vi "displayex.vi"(0 "EncMax":dbl[](array[numeric])=[6.50325, 6.5055000000000005, 6.4670000000000005], 1 "EncPos":cluster{"[0]":dbl, "[1]":dbl, "[2]":dbl}(graph)={"[0]"=1.92575, "[1]"=1.8495000000000001, "[2]"=4.599500000000001} caption="Position", 2 "TargetPos":dbl[](array[numeric])=[3.0, 3.0, 3.0], 3 "Blank":picture, 4 "CurrentState":enum16{"Initialize", "Run", "Finalize"}(ring)=enum."Run", 8 "HoldRange":dbl[](array[numeric])=[3.0, 3.0, 3.0]) -> (5 "Display":picture)   [LabVIEW 2011]
panel:
  in  "DispH":u32=870
  in  "PicRects":T1={"PicTar"={"Index"={"left"=0, "top"=325, "right"=0, "bottom"=525}, "Middle"={"left"=0, "top"=625, "right"=0, "bottom"=825}, "Thumb"={"left"=0, "top"=25, "right"=0, "bottom"=225}}, "PicPos"={"Index"={"left"=0, "top"=325, "right"=0, "bottom"=525}, "Middle"={"left"=0, "top"=625, "right"=0, "bottom"=825}, "Thumb"={"left"=0, "top"=25, "right"=0, "bottom"=225}}}
  in  "PicSizes":T2={"TarHeight"=200, "PosHeight"=200, "TarWidth"=200, "PosWidth"=200}
  in  "DispW":u32=1362
  in  "PosColor":cluster{"Index":u32, "Middle":u32, "Thumb":u32}={"Index"=11372, "Middle"=2113536, "Thumb"=7405568}
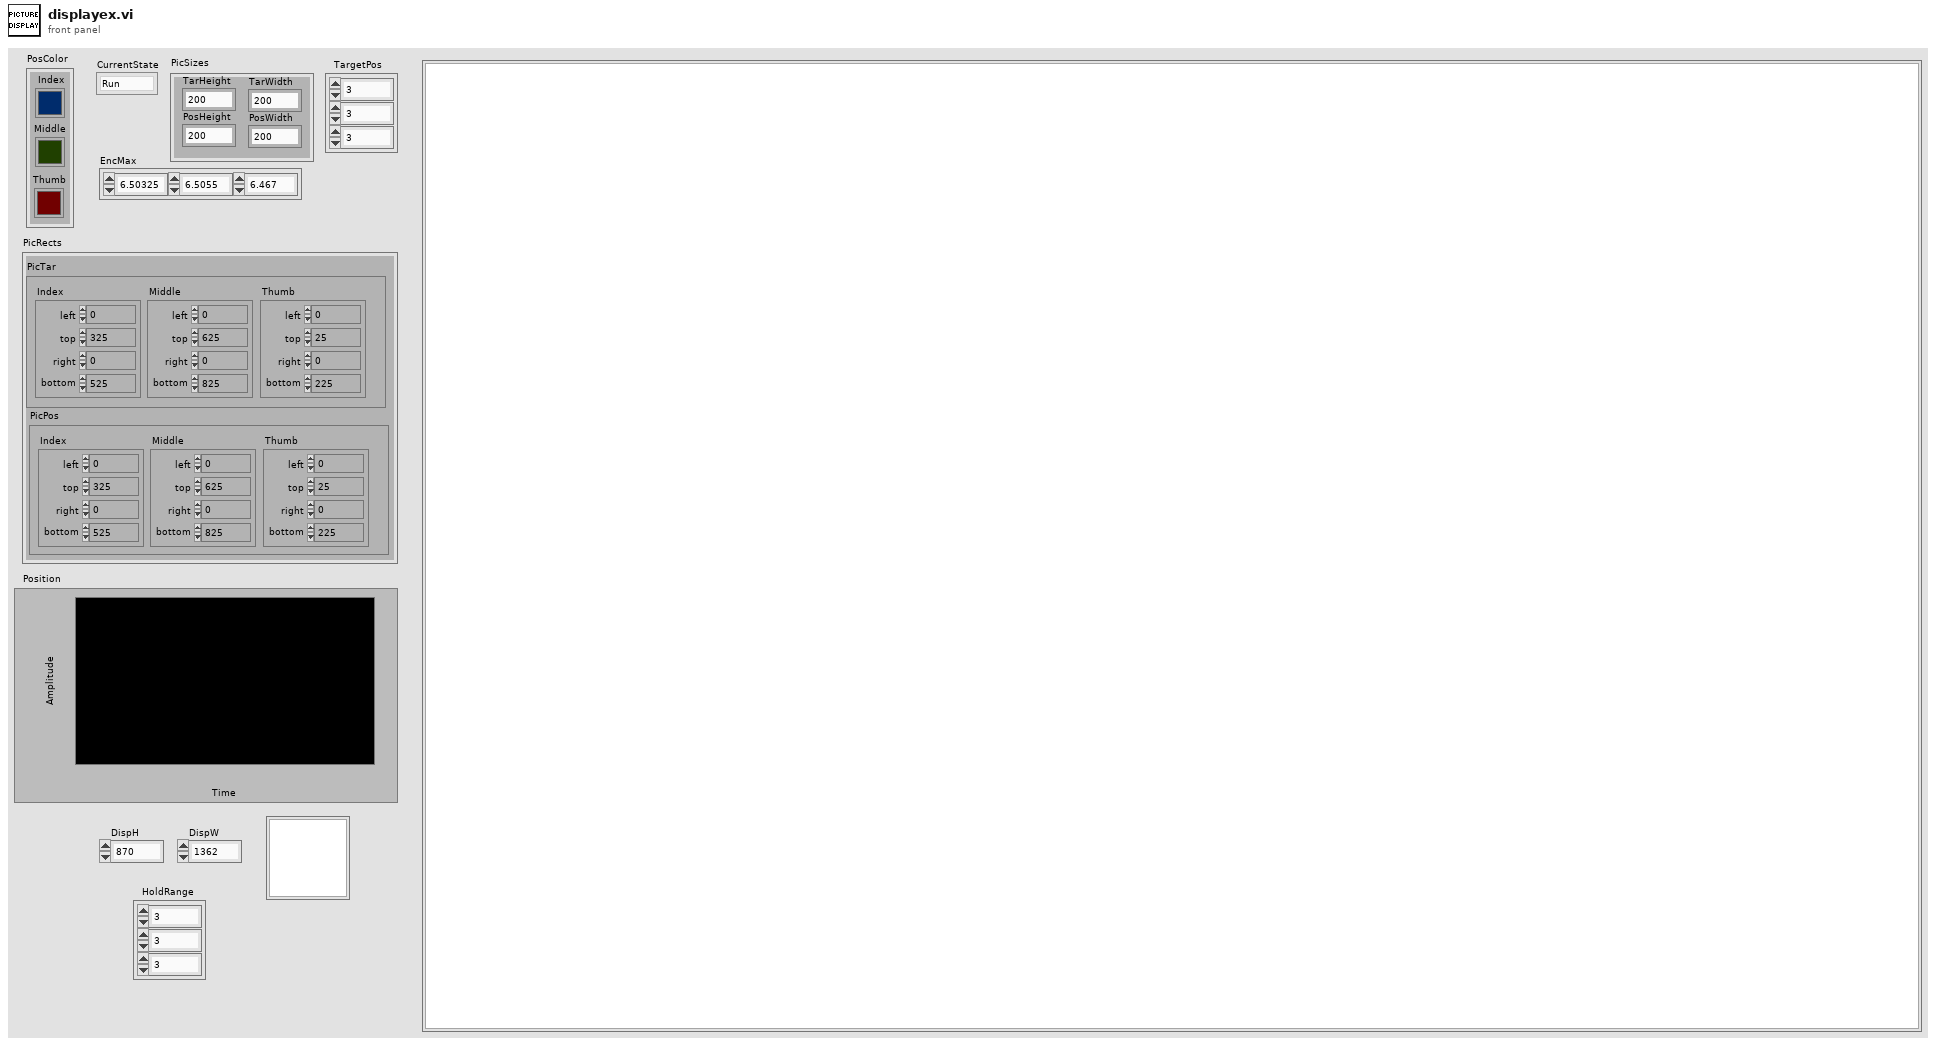
[diagram p1: front panel]
types:
  T1 = cluster{"PicTar":cluster{"Index":cluster{"left":i16, "top":i16, "right":i16, "bottom":i16}, "Middle":cluster{"left":i16, "top":i16, "right":i16, "bottom":i16}, "Thumb":cluster{"left":i16, "top":i16, "right":i16, "bottom":i16}}, "PicPos":cluster{"Index":cluster{"left":i16, "top":i16, "right":i16, "bottom":i16}, "Middle":cluster{"left":i16, "top":i16, "right":i16, "bottom":i16}, "Thumb":cluster{"left":i16, "top":i16, "right":i16, "bottom":i16}}}
  T2 = cluster{"TarHeight":i32, "PosHeight":i32, "TarWidth":i32, "PosWidth":i32}
  T3 = cluster{"Width":u16, "Style":enum32{"Solid", "Dash", "Dot", "DashDot", "DashDotDot"}}
  T4 = typedef "LVBoundsTypeDef.ctl" = cluster{"Width":u32, "Height":u32}
  T5 = cluster{"left":i16, "top":i16, "right":i16, "bottom":i16}
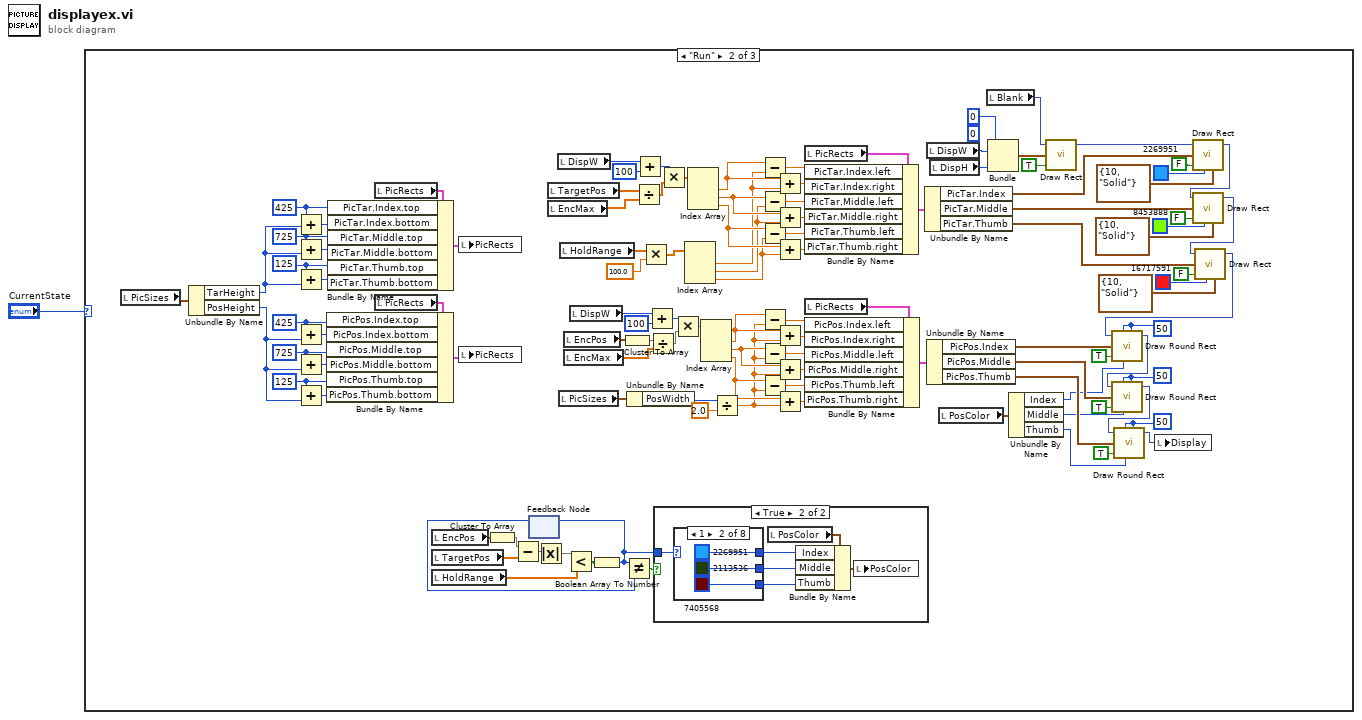
[diagram p0: block diagram]
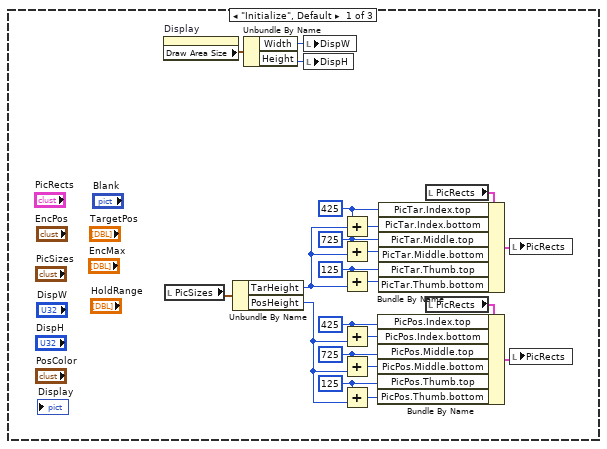
[diagram p2: hidden frame]
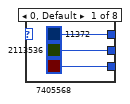
[diagram p4: hidden frame]
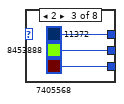
[diagram p5: hidden frame]
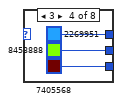
[diagram p6: hidden frame]
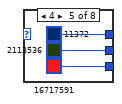
[diagram p7: hidden frame]
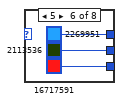
[diagram p8: hidden frame]
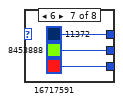
[diagram p9: hidden frame]
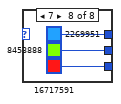
[diagram p10: hidden frame]
diagram:
  n1 = case shown="\"Run\"" "CurrentState" {
    frame "Initialize", Default {
      w15 = 125
      w18 = 725
      w13 = 425
      w11 = 125
      w21 = 725
      w8 = 425
      n2 = property on="Display" class="Pict"() -> ("Draw Area Size"=w4:T4)  [unwired: 2 in, 2 out]
      n3 = local read "PicSizes"() -> (w5:T2)
      n4 = Unbundle By Name(w5) -> ("TarHeight"=w6:i32, "PosHeight"=w7:i32)
      n5 = Unbundle By Name(w4) -> ("Width"=w3:u32, "Height"=w2:u32)
      n6 = local write "DispW"(w3) -> ()
      n7 = local write "DispH"(w2) -> ()
      n8 = Add(x=w13, y=w6) -> (x+y=w14:i32)
      n9 = Add(x=w18, y=w6) -> (x+y=w19:i32)
      n10 = Add(x=w15, y=w6) -> (x+y=w12:i32)
      n11 = Add(x=w8, y=w7) -> (x+y=w9:i32)
      n12 = Add(x=w21, y=w7) -> (x+y=w20:i32)
      n13 = Add(x=w11, y=w7) -> (x+y=w10:i32)
      n14 = local read "PicRects"() -> (w16:T1)
      n15 = Bundle By Name(cluster=w16, "PicTar.Index.top"=w13, "PicTar.Index.bottom"=w14, "PicTar.Middle.top"=w18, "PicTar.Middle.bottom"=w19, "PicTar.Thumb.top"=w15, "PicTar.Thumb.bottom"=w12) -> (w17:T1)
      n16 = local read "PicRects"() -> (w23:T1)
      n17 = Bundle By Name(cluster=w23, "PicPos.Index.top"=w8, "PicPos.Index.bottom"=w9, "PicPos.Middle.top"=w21, "PicPos.Middle.bottom"=w20, "PicPos.Thumb.top"=w11, "PicPos.Thumb.bottom"=w10) -> (w22:T1)
      n18 = local write "PicRects"(w17) -> ()
      n19 = local write "PicRects"(w22) -> ()
    }
    frame "Run" {
      w53 = 125
      w52 = 725
      w51 = 425
      w60 = 125
      w67 = 725
      w57 = 425
      w109 = i16 50 ("oval width")
      w110 = i16 50 ("oval width")
      w126 = i16 50 ("oval width")
      n20 = local read "PicSizes"() -> (w54:T2)
      n21 = Unbundle By Name(w54) -> ("TarHeight"=w55:i32, "PosHeight"=w56:i32)
      n22 = Add(x=w51, y=w55) -> (x+y=w62:i32)
      n23 = Add(x=w52, y=w55) -> (x+y=w65:i32)
      n24 = Add(x=w53, y=w55) -> (x+y=w61:i32)
      n25 = Add(x=w57, y=w56) -> (x+y=w58:i32)
      n26 = Add(x=w67, y=w56) -> (x+y=w66:i32)
      n27 = Add(x=w60, y=w56) -> (x+y=w59:i32)
      n28 = local read "PicRects"() -> (w63:T1)
      n29 = Bundle By Name(cluster=w63, "PicTar.Index.top"=w51, "PicTar.Index.bottom"=w62, "PicTar.Middle.top"=w52, "PicTar.Middle.bottom"=w65, "PicTar.Thumb.top"=w53, "PicTar.Thumb.bottom"=w61) -> (w64:T1)
      n30 = local read "PicRects"() -> (w69:T1)
      n31 = Bundle By Name(cluster=w69, "PicPos.Index.top"=w57, "PicPos.Index.bottom"=w58, "PicPos.Middle.top"=w67, "PicPos.Middle.bottom"=w66, "PicPos.Thumb.top"=w60, "PicPos.Thumb.bottom"=w59) -> (w68:T1)
      n32 = local read "EncPos"() -> (w90:cluster{"[0]":dbl, "[1]":dbl, "[2]":dbl})
      n33 = local read "TargetPos"() -> (w92:dbl[])
      n34 = local read "HoldRange"() -> (w24:dbl[])
      n35 = local write "PicRects"(w64) -> ()
      n36 = local write "PicRects"(w68) -> ()
      n37 = Cluster To Array(cluster=w90) -> (array=w91:dbl[])
      n38 = Subtract(x=w91, y=w92) -> (x-y=w93:dbl[])
      n39 = feedback #1() -> (w87:u32)  [unwired: 1 in]
      n40 = Absolute Value(x=w93) -> (abs(x)=w88:dbl[])
      n41 = local read "TargetPos"() -> (w96:dbl[])
      n42 = local read "EncMax"() -> (w37:dbl[])
      n43 = local read "DispW"() -> (w36:u32)
      n44 = local read "PicSizes"() -> (w103:T2)
      n45 = local read "HoldRange"() -> (w30:dbl[])
      n46 = local read "EncPos"() -> (w107:cluster{"[0]":dbl, "[1]":dbl, "[2]":dbl})
      n47 = local read "EncMax"() -> (w38:dbl[])
      n48 = Less?(x=w88, y=w24) -> (x < y?=w94:bool[])
      n49 = local read "DispW"() -> (w32:u32)
      n50 = Boolean Array To Number(Boolean array=w94) -> (number=w89:u32)
      n51 = feedback-in #1(w89) -> ()
      n52 = Cluster To Array(cluster=w107) -> (array=w106:dbl[])
      n53 = Not Equal?(x=w89, y=w87) -> (x != y?=w95:bool)
      n54 = Unbundle By Name(w103) -> ("PosWidth"=w40:i32)
      n55 = Divide(x=w96, y=w37) -> (x/y=w97:dbl[])
      n56 = Add(x=w36, y=u32 100) -> (x+y=w35:u32)
      n57 = Multiply(x=w30, y=100.0) -> (x*y=w28:dbl[])
      n58 = Add(x=w32, y=u32 100) -> (x+y=w31:u32)
      n59 = Divide(x=w106, y=w38) -> (x/y=w108:dbl[])
      n60 = case shown="True" w95 {
        tunnel: w89 -> [_ w144]
        frame False {
        }
        frame True {
          n61 = case shown="1" w144 {
            tunnel: [u32 11372 u32 2269951 u32 11372 u32 2269951 u32 11372 u32 2269951 u32 11372 u32 2269951] -> w142
            tunnel: [u32 2113536 u32 2113536 u32 8453888 u32 8453888 u32 2113536 u32 2113536 u32 8453888 u32 8453888] -> w141
            tunnel: [u32 7405568 u32 7405568 u32 7405568 u32 7405568 u32 16717591 u32 16717591 u32 16717591 u32 16717591] -> w140
            frame 0, Default {
            }
            frame 1 {
            }
            frame 2 {
            }
            frame 3 {
            }
            frame 4 {
            }
            frame 5 {
            }
            frame 6 {
            }
            frame 7 {
            }
          }
          n62 = local read "PosColor"() -> (w143:cluster{"Index":u32, "Middle":u32, "Thumb":u32})
          n63 = Bundle By Name(cluster=w143, "Index"=w142, "Middle"=w141, "Thumb"=w140) -> (w139:cluster{"Index":u32, "Middle":u32, "Thumb":u32})
          n64 = local write "PosColor"(w139) -> ()
        }
      }
      n65 = Multiply(x=w35, y=w97) -> (x*y=w98:dbl[])
      n66 = Multiply(x=w31, y=w108) -> (x*y=w105:dbl[])
      n67 = Index Array(array=w28) -> (element #1=w25:dbl, element #2=w26:dbl, element #3=w27:dbl)  [unwired: 3 in]
      n68 = Index Array(array=w98) -> (element #1=w83:dbl, element #2=w82:dbl, element #3=w81:dbl)  [unwired: 3 in]
      n69 = Index Array(array=w105) -> (element #1=w74:dbl, element #2=w73:dbl, element #3=w72:dbl)  [unwired: 3 in]
      n70 = Divide(x=w40, y=2.0) -> (x/y=w39:dbl)
      n71 = Subtract(x=w83, y=w25) -> (x-y=w85:dbl)
      n72 = Subtract(x=w82, y=w26) -> (x-y=w84:dbl)
      n73 = Subtract(x=w81, y=w27) -> (x-y=w86:dbl)
      n74 = Subtract(x=w74, y=w39) -> (x-y=w76:dbl)
      n75 = Subtract(x=w73, y=w39) -> (x-y=w75:dbl)
      n76 = Subtract(x=w72, y=w39) -> (x-y=w79:dbl)
      n77 = Add(x=w83, y=w25) -> (x+y=w101:dbl)
      n78 = Add(x=w82, y=w26) -> (x+y=w102:dbl)
      n79 = Add(x=w81, y=w27) -> (x+y=w100:dbl)
      n80 = Add(x=w74, y=w39) -> (x+y=w77:dbl)
      n81 = Add(x=w73, y=w39) -> (x+y=w78:dbl)
      n82 = Add(x=w72, y=w39) -> (x+y=w80:dbl)
      n83 = local read "PicRects"() -> (w99:T1)
      n84 = Bundle By Name(cluster=w99, "PicTar.Index.left"=w85, "PicTar.Index.right"=w101, "PicTar.Middle.left"=w84, "PicTar.Middle.right"=w102, "PicTar.Thumb.left"=w86, "PicTar.Thumb.right"=w100) -> (w70:T1)
      n85 = local read "PicRects"() -> (w104:T1)
      n86 = Bundle By Name(cluster=w104, "PicPos.Index.left"=w76, "PicPos.Index.right"=w77, "PicPos.Middle.left"=w75, "PicPos.Middle.right"=w78, "PicPos.Thumb.left"=w79, "PicPos.Thumb.right"=w80) -> (w71:T1)
      n87 = Unbundle By Name(w70) -> ("PicTar.Index"=w123:T5, "PicTar.Middle"=w122:T5, "PicTar.Thumb"=w121:T5)
      n88 = local read "DispW"() -> (w47:u32)
      n89 = Unbundle By Name(w71) -> ("PicPos.Index"=w117:T5, "PicPos.Middle"=w116:T5, "PicPos.Thumb"=w115:T5)
      n90 = local read "DispH"() -> (w46:u32)
      n91 = local read "PosColor"() -> (w114:cluster{"Index":u32, "Middle":u32, "Thumb":u32})
      n92 = local read "Blank"() -> (w43:picture)
      n93 = Bundle(0, 0, "DispW"=w47, "DispH"=w46) -> (w45:cluster{i32, i32, "DispW":u32, "DispH":u32})  [unwired: 1 in]
      n94 = Unbundle By Name(w114) -> ("Index"=w111:u32, "Middle"=w112:u32, "Thumb"=w113:u32)
      n95 = call <vilib>:"Draw Rect.vi"("picture"=w43, "rect"=w45, "fill?(F)"=TRUE) -> ("new picture"=w42:picture)  [unwired: 6 in]
      n96 = call <vilib>:"Draw Rect.vi"("picture"=w42, "rect"=w123, "fill?(F)"=FALSE, "color(black)"=u32 2269951, "pen"=T3 {"Width"=10, "Style"=enum."Solid"}) -> ("new picture"=w124:picture)  [unwired: 4 in]
      n97 = call <vilib>:"Draw Rect.vi"("picture"=w124, "rect"=w122, "fill?(F)"=FALSE, "color(black)"=u32 8453888, "pen"=T3 {"Width"=10, "Style"=enum."Solid"}) -> ("new picture"=w125:picture)  [unwired: 4 in]
      n98 = call <vilib>:"Draw Rect.vi"("picture"=w125, "rect"=w121, "fill?(F)"=FALSE, "color(black)"=u32 16717591, "pen"=T3 {"Width"=10, "Style"=enum."Solid"}) -> ("new picture"=w128:picture)  [unwired: 4 in]
      n99 = call <vilib>:"Draw Round Rect.vi"("picture"=w128, "oval width"=w126, "rect"=w117, "fill?(F)"=TRUE, "color(black)"=w111, "oval height"=w126) -> ("new picture"=w129:picture)  [unwired: 3 in]
      n100 = call <vilib>:"Draw Round Rect.vi"("picture"=w129, "oval width"=w110, "rect"=w116, "fill?(F)"=TRUE, "color(black)"=w112, "oval height"=w110) -> ("new picture"=w127:picture)  [unwired: 3 in]
      n101 = call <vilib>:"Draw Round Rect.vi"("picture"=w127, "oval width"=w109, "rect"=w115, "fill?(F)"=TRUE, "color(black)"=w113, "oval height"=w109) -> ("new picture"=w44:picture)  [unwired: 3 in]
      n102 = local write "Display"(w44) -> ()
    }
    frame "Finalize" {
    }
  }
